vi "Begin.vi"(8 "error in":errorcluster) -> (0 "error out":errorcluster)   [LabVIEW 2020]
doc: "Called before other user functions, this VI can be used to open I/O refnums, load in file data, and do general program initialization. Notice that the <B>error out</B> terminal is simply used for data flow. Wiring it to other structures or subVIs ensures that this VI runs first."
uses:
  <vilib>/Rock Robotics/WPI/DriverStation/WPI_DriverStationRobotMode2.ctl
  <vilib>/Rock Robotics/WPI/Joystick/WPI_JoystickDeviceEnum.ctl
  Robot Global Data.vi
  <vilib>/Rock Robotics/Network Tables/NT Write String Array.vi
  <vilib>/Rock Robotics/SystemInterfaces/DIO/FPGA_DIOPWMChannel.ctl
  <vilib>/Rock Robotics/WPI/ThirdParty/Phoenix-LabVIEW/Motor Controller/Closed Loop/Motion Profile/CTRE_Phoenix_MotorControl_BufferedTrajectoryPointStream_WriteAll.vi
  <vilib>/Rock Robotics/WPI/ThirdParty/Phoenix-LabVIEW/Motor Controller/Controls/CTRE_Phoenix_MotorControl_MotionProfileTrajectoryPoint.ctl
panel:
  out "Motion Profile Trajectory Point Array left":T1[](array[typedef])
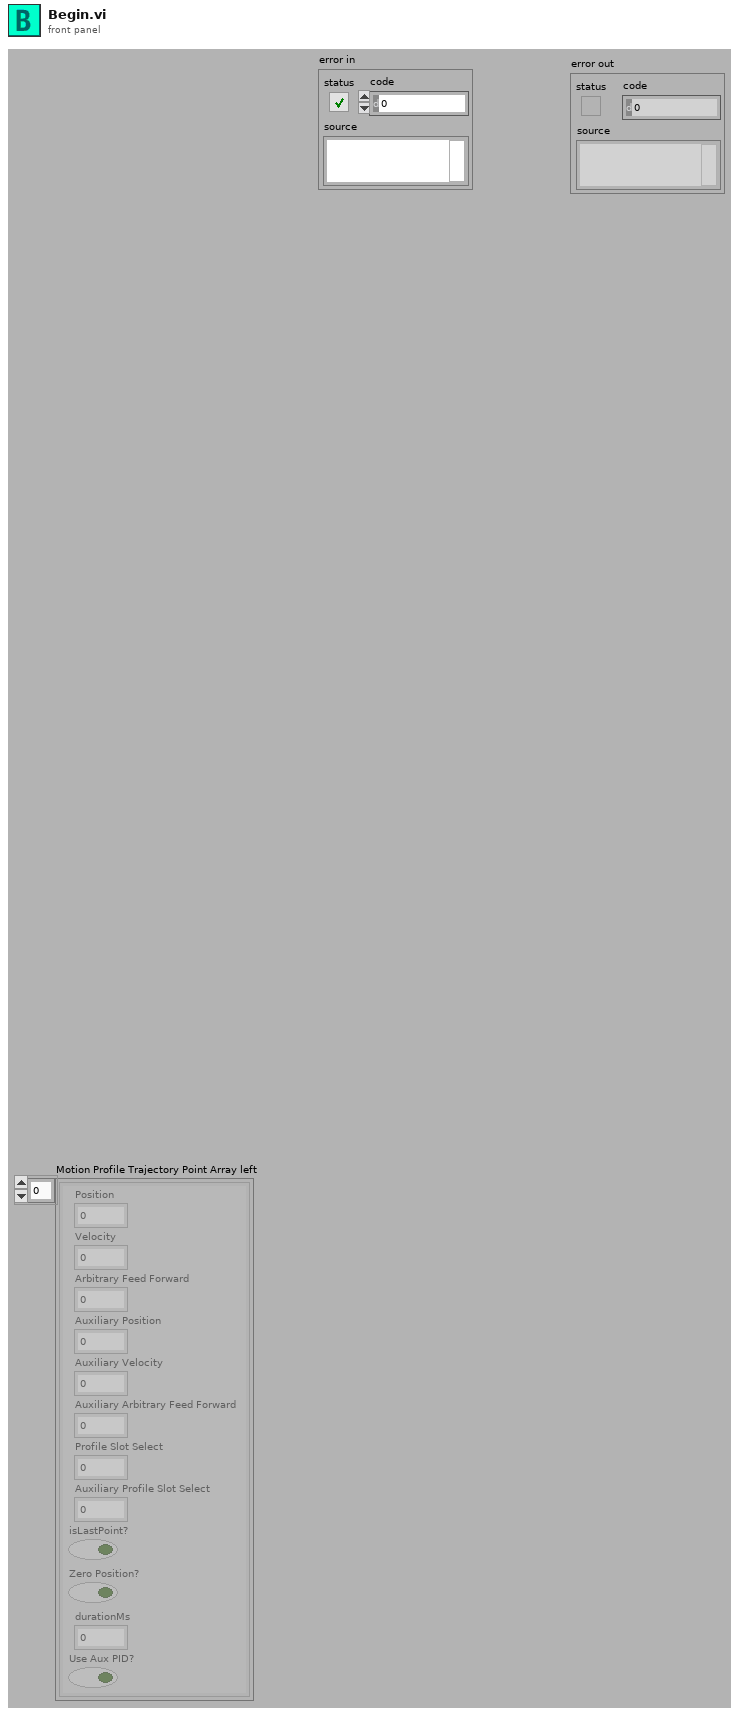
[diagram p1: front panel]
types:
  T1 = typedef "CTRE_Phoenix_MotorControl_MotionProfileTrajectoryPoint.ctl" = cluster{"Position":dbl, "Velocity":dbl, "Arbitrary Feed Forward":dbl, "Auxiliary Position":dbl, "Auxiliary Velocity":dbl, "Auxiliary Arbitrary Feed Forward":dbl, "Profile Slot Select":i32, "Auxiliary Profile Slot Select":i32, "isLastPoint?":bool, "Zero Position?":bool, "durationMs":u32, "Use Aux PID?":bool}
  T2 = typedef "WPI_JoystickDeviceEnum.ctl" = enum16{"USB 0", "USB 1", "USB 2", "USB 3", "USB 4", "USB 5"}
  T3 = typedef "WPI_DriverStationRobotMode2.ctl" = enum16{"Autonomous Disabled", "Autonomous Enabled", "Teleop Disabled", "Teleop Enabled", "Disconnected", "Finish", "Test Disabled", "Test Enabled", "Emergency Stopped"}
  T4 = typedef "FPGA_DIOPWMChannel.ctl" = enum8{"PWM 0", "PWM 1", "PWM 2", "PWM 3", "PWM 4", "PWM 5", "PWM 6", "PWM 7", "PWM 8", "PWM 9", "PWM MXP 0", "PWM MXP 1", "PWM MXP 2", "PWM MXP 3", "PWM MXP 4", "PWM MXP 5", "PWM MXP 6", "PWM MXP 7", "PWM MXP 8", "PWM MXP 9", "Invalid"}
  T5 = typedef "WPI_ServoDeviceRef.ctl" = cluster{"DeviceStatus":errorcluster, "PWM Channel":T4, "DeadBand":T6}
  T6 = typedef "WPI_PWMDeadband.ctl" = cluster{"Name":string, "maxPositivePwm":i32, "minPositivePwm":i32, "centerPwm":i32, "maxNegativePwm":i32, "minNegativePwm":i32, "angularRange":u16}
  T7 = typedef "WPI_MotorControlDeviceRef.ctl" = cluster{"DeviceStatus":errorcluster, "Type":T8, "PWM":cluster{"PWM Channel":T4, "DeadBand":T6}, "CAN":cluster{"Device Number":u8, "SetOutput VI Ref":variant, "GetOutput VI Ref":variant, "Enable VI Ref":variant, "Disable VI Ref":variant, "Data":variant}, "Invert":bool, "DIO PWM":cluster{"PWM \"Enable\" Channel":T4, "DIOChannel":T9, "PWM Rate":dbl}}
  T8 = typedef "WPI_MotorControlType.ctl" = enum16{"PWM", "CAN", "DIO PWM"}
  T9 = typedef "FPGA_DIOChannel.ctl" = enum8{"DIO 0", "DIO 1", "DIO 2", "DIO 3", "DIO 4", "DIO 5", "DIO 6", "DIO 7", "DIO 8", "DIO 9", "DIO MXP 0", "DIO MXP 1", "DIO MXP 2", "DIO MXP 3", "DIO MXP 4", "DIO MXP 5", "DIO MXP 6", "DIO MXP 7", "DIO MXP 8", "DIO MXP 9", "DIO MXP 10", "DIO MXP 11", "DIO MXP 12", "DIO MXP 13", "DIO MXP 14", "DIO MXP 15", "SPI Port CS1", "SPI Port CS2", "SPI Port CS3", "SPI Port MISO", "SPI Port MOSI", "Invalid"}
  T10 = typedef "WPI_JoystickDevRef.ctl" = cluster{"Device":T2}
  T11 = typedef "CTRE_Phoenix_MotorControl_BufferedTrajectoryPointStream_DeviceRef.ctl" = cluster{"Handle":u64, "Library Path":path}
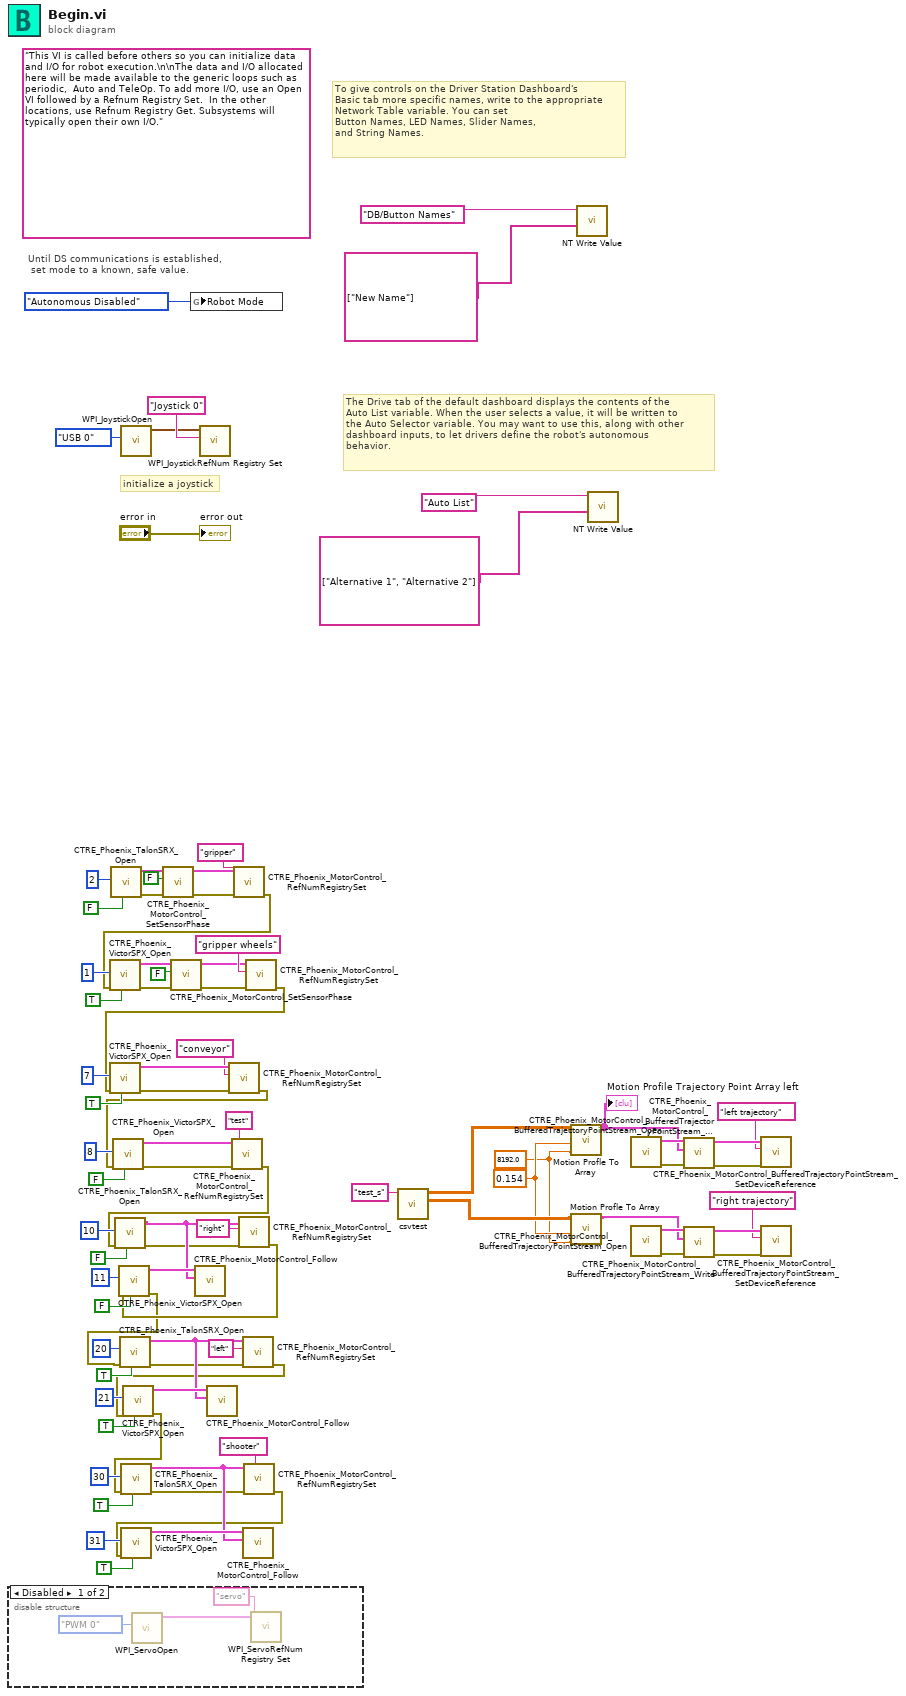
[diagram p0: block diagram]
diagram:
  w2 = 8192.0 ("Encoder Units")
  w3 = 0.154 ("Wheel Diameter (M)")
  (unwired) "This VI is called before others so you can initialize data and I/O for robot execution.\n\nThe data and I/O allocated here will be made available to the generic loops such as periodic,  Auto and TeleOp. To add more I/O, use an Open VI followed by a Refnum Registry Set.  In the other locations, use Refnum Registry Get. Subsystems will typically open their own I/O."
  # "The Drive tab of the default dashboard displays the contents of the\nAuto List variable. When the user selects a value, it will be written to\nthe Auto Selector variable. You may want to use this, along with other\ndashboard inputs, to let drivers define the robot's autonomous\nbehavior."
  # "To give controls on the Driver Station Dashboard's\nBasic tab more specific names, write to the appropriate\nNetwork Table variable. You can set\nButton Names, LED Names, Slider Names,\nand String Names."
  # "initialize a joystick"
  # "Until DS communications is established,\n set mode to a known, safe value."
  n1 = disable-structure shown="Disabled" {
    frame Disabled {
      n2 = call <vilib>:"WPI_ServoOpen.vi"("PWM Channel"=FPGA_DIOPWMChannel."PWM 0") -> ("ServoDeviceRef"=w87:T5)  [unwired: 9 in, 1 out]
      n3 = call <vilib>:"WPI_ServoRefNum Registry Set.vi"("refnum name"="servo", "ServoDeviceRef"=w87) -> ()  [unwired: 8 in, 2 out]
    }
    frame Enabled {
    }
  }
  n4 = call <vilib>:"CTRE_Phoenix_TalonSRX_Open.vi"("Invert"=FALSE, "Device Number"=u8 2) -> ("error out"=w36:errorcluster, "PhoenixMotorControlDevRef"=w35:T7)  [unwired: 8 in]
  n5 = call <vilib>:"WPI_JoystickOpen.vi"("JoystickDevice"=WPI_JoystickDeviceEnum."USB 0") -> ("JoystickDevRef"=w83:T10)  [unwired: 10 in]
  n6 = call <vilib>:"CTRE_Phoenix_MotorControl_SetSensorPhase.vi"("error in (no error)"=w36, "PhaseSensor"=FALSE, "PhoenixMotorControlDevRef"=w35) -> ("error out"=w32:errorcluster, "PhoenixMotorControlDevRef"=w34:T7)  [unwired: 7 in]
  n7 = global write "Robot Global Data.vi" "Robot Mode"(WPI_DriverStationRobotMode2."Autonomous Disabled" ("Robot Mode")) -> ()
  n8 = call <vilib>:"WPI_JoystickRefNum Registry Set.vi"("refnum name"="Joystick 0", "JoystickDevRef"=w83) -> ()  [unwired: 8 in, 2 out]
  n9 = call <vilib>:"CTRE_Phoenix_MotorControl_RefNumRegistrySet.vi"("error in (no error)"=w32, "refnum name"="gripper", "PhoenixMotorControlDevRef"=w34) -> ("error out"=w31:errorcluster)  [unwired: 7 in, 1 out]
  n10 = call <vilib>:"CTRE_Phoenix_VictorSPX_Open.vi"("Invert"=TRUE, "error in"=w31, "Device Number"=u8 1) -> ("error out"=w41:errorcluster, "PhoenixMotorControlDevRef"=w40:T7)  [unwired: 7 in]
  n11 = call <vilib>:"CTRE_Phoenix_MotorControl_SetSensorPhase.vi"("error in (no error)"=w41, "PhaseSensor"=FALSE, "PhoenixMotorControlDevRef"=w40) -> ("error out"=w38:errorcluster, "PhoenixMotorControlDevRef"=w37:T7)  [unwired: 7 in]
  n12 = call <vilib>:"CTRE_Phoenix_MotorControl_RefNumRegistrySet.vi"("error in (no error)"=w38, "refnum name"="gripper wheels", "PhoenixMotorControlDevRef"=w37) -> ("error out"=w30:errorcluster)  [unwired: 7 in, 1 out]
  n13 = call <vilib>:"CTRE_Phoenix_VictorSPX_Open.vi"("Invert"=TRUE, "error in"=w30, "Device Number"=u8 7) -> ("error out"=w29:errorcluster, "PhoenixMotorControlDevRef"=w53:T7)  [unwired: 7 in]
  n14 = call <vilib>:"CTRE_Phoenix_MotorControl_RefNumRegistrySet.vi"("error in (no error)"=w29, "refnum name"="conveyor", "PhoenixMotorControlDevRef"=w53) -> ("error out"=w28:errorcluster)  [unwired: 7 in, 1 out]
  n15 = call <vilib>:"CTRE_Phoenix_VictorSPX_Open.vi"("Invert"=FALSE, "error in"=w28, "Device Number"=u8 8) -> ("error out"=w27:errorcluster, "PhoenixMotorControlDevRef"=w43:T7)  [unwired: 7 in]
  n16 = call <vilib>:"CTRE_Phoenix_MotorControl_RefNumRegistrySet.vi"("error in (no error)"=w27, "refnum name"="test", "PhoenixMotorControlDevRef"=w43) -> ("error out"=w26:errorcluster)  [unwired: 7 in, 1 out]
  n17 = call <vilib>:"CTRE_Phoenix_TalonSRX_Open.vi"("Invert"=FALSE, "error in"=w26, "Device Number"=u8 10) -> ("error out"=w25:errorcluster, "PhoenixMotorControlDevRef"=w72:T7)  [unwired: 7 in]
  n18 = call <vilib>:"CTRE_Phoenix_MotorControl_RefNumRegistrySet.vi"("error in (no error)"=w25, "refnum name"="right", "PhoenixMotorControlDevRef"=w72) -> ("error out"=w24:errorcluster)  [unwired: 7 in, 1 out]
  n19 = call <vilib>:"CTRE_Phoenix_VictorSPX_Open.vi"("Invert"=FALSE, "error in"=w24, "Device Number"=u8 11) -> ("error out"=w23:errorcluster, "PhoenixMotorControlDevRef"=w76:T7)  [unwired: 7 in]
  n20 = call <vilib>:"CTRE_Phoenix_TalonSRX_Open.vi"("Invert"=TRUE, "error in"=w23, "Device Number"=u8 20) -> ("error out"=w22:errorcluster, "PhoenixMotorControlDevRef"=w61:T7)  [unwired: 7 in]
  n21 = call <vilib>:"CTRE_Phoenix_MotorControl_Follow.vi"("Master Controller to Follow"=w72, "PhoenixMotorControlDevRef"=w76) -> ()  [unwired: 8 in, 2 out]
  n22 = call <vilib>:"CTRE_Phoenix_MotorControl_RefNumRegistrySet.vi"("error in (no error)"=w22, "refnum name"="left", "PhoenixMotorControlDevRef"=w61) -> ("error out"=w21:errorcluster)  [unwired: 7 in, 1 out]
  n23 = call <vilib>:"CTRE_Phoenix_VictorSPX_Open.vi"("Invert"=TRUE, "error in"=w21, "Device Number"=u8 21) -> ("error out"=w20:errorcluster, "PhoenixMotorControlDevRef"=w75:T7)  [unwired: 7 in]
  n24 = call <vilib>:"CTRE_Phoenix_TalonSRX_Open.vi"("Invert"=TRUE, "error in"=w20, "Device Number"=u8 30) -> ("error out"=w19:errorcluster, "PhoenixMotorControlDevRef"=w57:T7)  [unwired: 7 in]
  n25 = call <vilib>:"CTRE_Phoenix_MotorControl_Follow.vi"("Master Controller to Follow"=w61, "PhoenixMotorControlDevRef"=w75) -> ()  [unwired: 8 in, 2 out]
  n26 = call <vilib>:"CTRE_Phoenix_MotorControl_RefNumRegistrySet.vi"("error in (no error)"=w19, "refnum name"="shooter", "PhoenixMotorControlDevRef"=w57) -> ("error out"=w18:errorcluster)  [unwired: 7 in, 1 out]
  n27 = call <vilib>:"CTRE_Phoenix_VictorSPX_Open.vi"("Invert"=TRUE, "error in"=w18, "Device Number"=u8 31) -> ("PhoenixMotorControlDevRef"=w62:T7)  [unwired: 7 in, 1 out]
  n28 = call <vilib>:"CTRE_Phoenix_MotorControl_Follow.vi"("Master Controller to Follow"=w57, "PhoenixMotorControlDevRef"=w62) -> ()  [unwired: 8 in, 2 out]
  n29 = call "csvtest.vi"("path name"="test_s") -> ("right path"=w5:dbl[][], "left path"=w6:dbl[][])  [unwired: 9 in]
  n30 = call "Motion Profle To Array.vi"("Encoder Units"=w2, "Wheel Diameter (M)"=w3, "path"=w6) -> ("Motion Profile Trajectory Point Array"=w1:T1[])  [unwired: 8 in]
  "Motion Profile Trajectory Point Array left" <- w1
  n31 = call "Motion Profle To Array.vi"("Encoder Units"=w2, "Wheel Diameter (M)"=w3, "path"=w5) -> ("Motion Profile Trajectory Point Array"=w4:T1[])  [unwired: 8 in]
  n32 = call-poly <vilib>:"NT Write Value.vi"("String Array"=string[] ["New Name"], "Name"="DB/Button Names") -> ()  [unwired: 9 in, 1 out]
  n33 = call-poly <vilib>:"NT Write Value.vi"("String Array"=string[] ["Alternative 1", "Alternative 2"], "Name"="Auto List") -> ()  [unwired: 9 in, 1 out]
  n34 = call <vilib>:"CTRE_Phoenix_MotorControl_BufferedTrajectoryPointStream_Open.vi"() -> ("error out"=w16:errorcluster, "BufferedTrajectoryPointStream_DevRef"=w15:T11)  [unwired: 10 in]
  n35 = call <vilib>:"CTRE_Phoenix_MotorControl_BufferedTrajectoryPointStream_Open.vi"() -> ("error out"=w8:errorcluster, "BufferedTrajectoryPointStream_DevRef"=w9:T11)  [unwired: 10 in]
  n36 = call-poly <vilib>:"CTRE_Phoenix_MotorControl_BufferedTrajectoryPointStream_Write.vi"("error in"=w16, "Motion Profile Trajectory Point Array"=w1, "BufferedTrajectoryPointStream_DevRef"=w15) -> ("error out"=w14:errorcluster, "BufferedTrajectoryPointStream_DevRef"=w13:T11)  [unwired: 7 in]
  n37 = call-poly <vilib>:"CTRE_Phoenix_MotorControl_BufferedTrajectoryPointStream_Write.vi"("error in"=w8, "Motion Profile Trajectory Point Array"=w4, "BufferedTrajectoryPointStream_DevRef"=w9) -> ("error out"=w10:errorcluster, "BufferedTrajectoryPointStream_DevRef"=w11:T11)  [unwired: 7 in]
  n38 = call <vilib>:"CTRE_Phoenix_MotorControl_BufferedTrajectoryPointStream_SetDeviceReference.vi"("error in (no error)"=w14, "refnum name"="left trajectory", "BufferedTrajectoryPointStream_DevRef"=w13) -> ()  [unwired: 7 in, 2 out]
  n39 = call <vilib>:"CTRE_Phoenix_MotorControl_BufferedTrajectoryPointStream_SetDeviceReference.vi"("error in (no error)"=w10, "refnum name"="right trajectory", "BufferedTrajectoryPointStream_DevRef"=w11) -> ()  [unwired: 7 in, 2 out]
  "error out" <- "error in"
